vi "Przenies enkodery FVG.vi"(7 "Akcja (Get)":T2, 8 "error in (no error)":errorcluster, 9 "Kana³ in":T1, 10 "dT in":dbl format="%#_13g", 11 "Zerowanie in":bool) -> (0 "error out":errorcluster, 1 "Kana³ out":T1, 2 "dT out":dbl format="%#_13g", 3 "Zerowanie out":bool)   [LabVIEW 2013]
doc: "Przenosi ustawienia enkodera z pêtli gui do pêtli akwizycja"
uses:
  Kontrolki/FVGs/FVG akcje podstawowa.ctl
  Kontrolki/GUI/Encoder_chanel.ctl
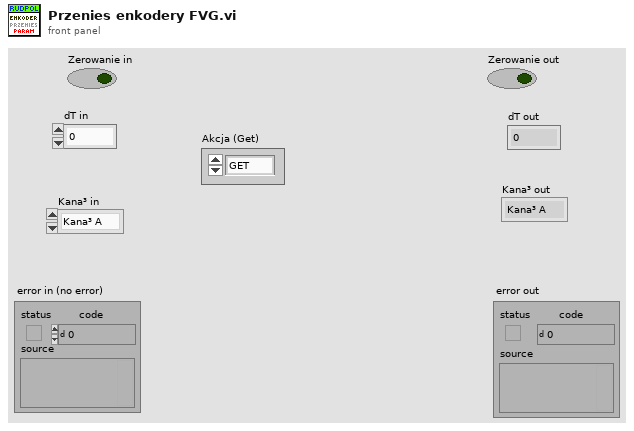
[diagram p1: front panel]
types:
  T1 = typedef "Encoder_chanel.ctl" = enum16{"Kana³ A", "Kana³ B"}
  T2 = typedef "FVG akcje podstawowa.ctl" = enum16{"GET", "SET"}
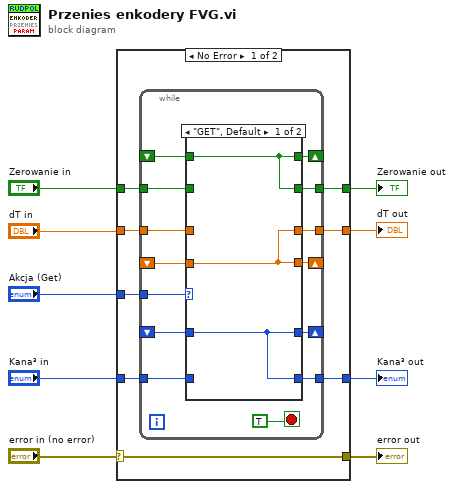
[diagram p0: block diagram]
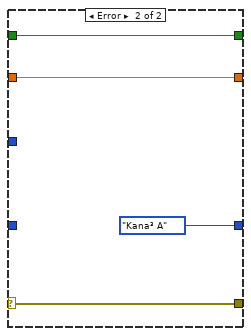
[diagram p3: hidden frame]
diagram:
  n1 = case shown="No Error" "error in (no error)" {
    selector: "error in (no error)" -> [w17 w41]
    tunnel: [w17 w41] -> w9
    tunnel: "Akcja (Get)" -> [w16 _]
    tunnel: "Kana³ in" -> [w15 _]
    tunnel: [w14 Encoder_chanel."Kana³ A" ("Kana³ in")] -> w1
    tunnel: "dT in" -> [w13 w39]
    tunnel: [w12 w39] -> w2
    tunnel: "Zerowanie in" -> [w11 w38]
    tunnel: [w10 w38] -> w3
    frame No Error {
      n2 = while {
        tunnel: w16 -> [w30]
        tunnel: w15 -> [w29]
        shift-right: [w28] -> _
        shift-left: _ -> [w27]
        tunnel: [w26] -> w14
        tunnel: w13 -> [w25]
        shift-right: [w24] -> _
        shift-left: _ -> [w22]
        tunnel: [w23] -> w12
        tunnel: w11 -> [w21]
        tunnel: [w20] -> w10
        shift-right: [w19] -> _
        shift-left: _ -> [w18]
        stop <- TRUE stop-if-true
        n3 = case shown="\"GET\", Default" w30 {
          tunnel: w29 -> [_ w37]
          tunnel: [w34 w37] -> w28
          tunnel: w27 -> [w34 _]
          tunnel: [w34 w37] -> w26
          tunnel: w25 -> [_ w36]
          tunnel: [w33 w36] -> w24
          tunnel: [w33 w36] -> w23
          tunnel: w22 -> [w33 _]
          tunnel: w21 -> [_ w35]
          tunnel: [w32 w35] -> w20
          tunnel: [w32 w35] -> w19
          tunnel: w18 -> [w32 _]
          frame "GET", Default {
          }
          frame "SET" {
          }
        }
      }
    }
    frame Error {
    }
  }
  "error out" <- w9
  "Zerowanie out" <- w3
  "dT out" <- w2
  "Kana³ out" <- w1
